vi "(SubVI)_Biuld_X_Y_for2DPSF.vi"(2 "X-Y Parameters":T1) -> (0 "X-Y Array":dbl[][](array[numeric]))   [LabVIEW 2019]
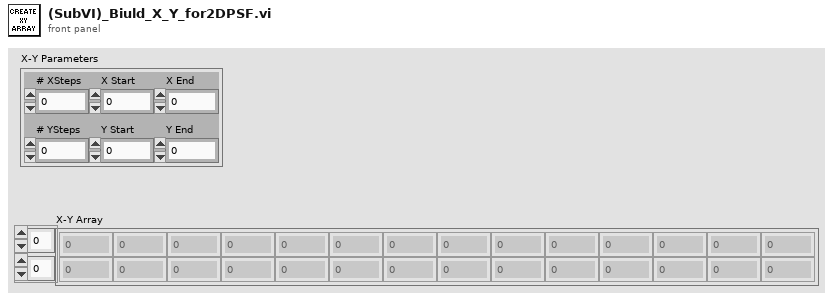
[diagram p1: front panel]
types:
  T1 = cluster{"# XSteps":dbl, "# YSteps":dbl, "X Start":dbl, "Y Start":dbl, "X End":dbl, "Y End":dbl}
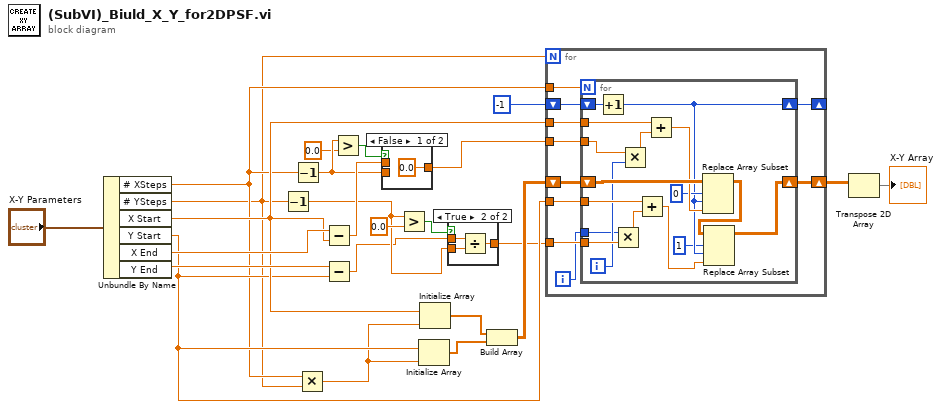
[diagram p0: block diagram]
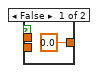
[diagram p2: hidden frame]
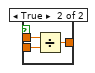
[diagram p3: hidden frame]
diagram:
  n1 = Unbundle By Name("X-Y Parameters") -> ("# XSteps"=w3:dbl, "# YSteps"=w2:dbl, "X Start"=w20:dbl, "Y Start"=w19:dbl, "X End"=w23:dbl, "Y End"=w22:dbl)
  n2 = Decrement(x=w2) -> (x-1=w5:dbl)
  n3 = Decrement(x=w3) -> (x-1=w10:dbl)
  n4 = Multiply(x=w3, y=w2) -> (x*y=w18:dbl)
  n5 = Subtract(x=w23, y=w20) -> (x-y=w21:dbl)
  n6 = Subtract(x=w22, y=w19) -> (x-y=w4:dbl)
  n7 = Greater?(x=w10, y=0.0) -> (0:w11:bool)
  n8 = case shown="False" w11 {
    tunnel: w21 -> [_ w28]
    tunnel: w10 -> [_ w27]
    tunnel: [0.0 w26] -> w13
    frame False {
    }
    frame True {
      n9 = Divide(x=w28, y=w27) -> (x/y=w26:dbl)
    }
  }
  n10 = Greater?(x=w5, y=0.0) -> (0:w8:bool)
  n11 = Initialize Array(w19, w18) -> (w16:dbl[])
  n12 = Initialize Array(w20, w18) -> (w17:dbl[])
  n13 = case shown="True" w8 {
    tunnel: w4 -> [_ w32]
    tunnel: w5 -> [_ w31]
    tunnel: [0.0 w30] -> w6
    frame False {
    }
    frame True {
      n14 = Divide(x=w32, y=w31) -> (x/y=w30:dbl)
    }
  }
  n15 = Build Array(w17, w16) -> (w15:dbl[][])
  n16 = for {
    N: w2 -> [_]
    tunnel: w3 -> [w42]
    tunnel: w20 -> [w41]
    tunnel: w19 -> [w40]
    shift-right: [w38] -> w12
    shift-left: w15 -> [w39]
    shift-right: [w36] -> _
    shift-left: -1 -> [w37]
    tunnel: w13 -> [w35]
    tunnel: w6 -> [w34]
    i -> [w33]
    n17 = for {
      N: w42 -> [_]
      tunnel: w41 -> [w56]
      tunnel: w40 -> [w50]
      shift-right: [w48] -> w38
      shift-left: w39 -> [w58]
      shift-right: [w46] -> w36
      shift-left: w37 -> [w59]
      tunnel: w35 -> [w57]
      tunnel: w34 -> [w51]
      tunnel: w33 -> [w43]
      i -> [w44]
      n18 = Increment(x=w59) -> (x+1=w46:i32)
      n19 = Multiply(x=w43, y=w51) -> (x*y=w52:dbl)
      n20 = Multiply(x=w57, y=w44) -> (x*y=w55:dbl)
      n21 = Add(x=w50, y=w52) -> (x+y=w49:dbl)
      n22 = Add(x=w56, y=w55) -> (x+y=w54:dbl)
      n23 = Replace Array Subset(array=w58, new element=w54, index (row)=0 ("disabled index (col)"), index (col)=w46) -> (w53:dbl[][])
      n24 = Replace Array Subset(array=w53, new element=w49, index (row)=1 ("disabled index (col)"), index (col)=w46) -> (w48:dbl[][])
    }
  }
  n25 = Transpose 2D Array(2D array=w12) -> (transposed array=→"X-Y Array":dbl[][])
